vi "Inputs.vi"(8 "error in (no error)":errorcluster, 11 "State in":T1={"State"=enum."Idle", "Start Time"=timestamp(0 s since 1904-01-01), "Configuration"={"Cycle Period"=0.0, "Ismatech"={"VISA resource name"="", "Simulated?"=FALSE, "Pump Number"=1.0, "Reverse?"=FALSE}, "Masterflex"={"VISA resource name"="", "Simulated?"=FALSE, "Pump Number"=1.0, "Reverse?"=FALSE}, "Mettler"={"VISA resource name"="", "Simulated?"=FALSE}, "Bronkhorst M13 Flow Meter"={"VISA resource name"="", "Simulated?"=FALSE, "Smoothing Steps"=1}, "PID 2 Parameters"={"Input Device"=enum."Bronkhorst M13", "Output Device"=enum."Ismatec ISM 831C", "Setpoint"=0.0, "PID gains"={"proportional gain (Kc)"=1.0, "integral time (Ti, min)"=0.01, "derivative time (Td, min)"=0.0}}, "Manual Entry"=0.0, "Auto?"=TRUE, "PID range"={"PID High"=100.0, "PID Low"=0.0, "High Warning"=100.0}, "Tacmina Settings"={"Analog DAQ Task"="", "Digital DAQ Task"=""}, "KNF SIMDOS Settings"={"VISA resource name"="", "Simulated?"=TRUE}, "ASIA Pump C"={"ASIA Pump #"=0, "channel"=0, "Simulated"=FALSE}, "VICI Settings"={"VISA resource name"="", "Pump ID"="", "Pump Head Vol"=0.0, "Reverse?"=FALSE, "Simulated?"=FALSE}, "FLOM Settings"={"VISA resource name"="", "Simulated?"=TRUE, "Pump Number"=0.0}, "SSI PR/LD Settings"={"VISA resource name"="", "Simulated?"=FALSE}, "Masterflex 75211 Settings"={"Analog DAQ Task"="", "Digital DAQ Task"=""}, "SSI P40 Settings"={"VISA resource name"="", "Simulated?"=TRUE}, "Ismatech 3 Channel Settings"={"VISA resource name"="", "Pump Number"=1, "Channel Number"=0, "Simulated?"=TRUE, "Reverse?"=FALSE}, "Bronkhorst M14 Settings"={"VISA resource name"="", "Simulated?"=FALSE, "Smoothing Steps"=1}, "Reset Totalizer"=FALSE, "Input Num Alarm Settings"=[], "Control Type"=enum."g/min"}, "Current Time"=timestamp(0 s since 1904-01-01), "PID 1 Parameters"={"Setpoint"=0.0, "PID gains"={"proportional gain (Kc)"=1.0, "integral time (Ti, min)"=0.01, "derivative time (Td, min)"=0.0}}, "First Iteration"=FALSE, "Data"={"Flowmeter (g/min)"=0.0, "Flowmeter (ml/min)"=0.0, "Density"=0.0, "FL Temp"=0.0, "Scale Output (g)"=0.0, "Scale Rate of Change (g/min)"=0.0, "PID 1 Output"=0.0, "PID 2 Process Variable"=0.0, "PID 2 output"=0.0, "Pump Flow"=0.0, "Pump Pressure"=0.0, "Totalized Value"=0.0}, "Process Name"="", "Pump On?"=enum."Off", "Input Error"=FALSE, "Output Error"=FALSE, "Log Started"=FALSE, "PID Overshoot"=FALSE, "Current Setpoint"=0.0} {"PID 1 Parameters"."PID gains"."derivative time (Td, min)" format="%.3f"; "PID 1 Parameters"."PID gains"."integral time (Ti, min)" format="%.3f"; "PID 1 Parameters"."PID gains"."proportional gain (Kc)" format="%.3f"; "Configuration"."Bronkhorst M14 Settings"."Smoothing Steps" min=1 step=1; "Configuration"."Ismatech 3 Channel Settings"."Channel Number" min=0 max=3; "Configuration"."Ismatech 3 Channel Settings"."Pump Number" min=1; "Configuration"."PID range"."PID Low" min=0.0 max=100.0 format="%.2f"; "Configuration"."PID range"."PID High" format="%.2f"; "Configuration"."PID 2 Parameters"."PID gains"."derivative time (Td, min)" format="%.3f"; "Configuration"."PID 2 Parameters"."PID gains"."integral time (Ti, min)" format="%.3f"; "Configuration"."PID 2 Parameters"."PID gains"."proportional gain (Kc)" format="%.3f"; "Configuration"."Bronkhorst M13 Flow Meter"."Smoothing Steps" min=1 step=1; "Configuration"."ASIA Pump C"."channel" min=0 max=1 step=1; "Configuration"."Ismatech"."Pump Number" min=1.0 max=20.0 step=1.0; "Configuration"."Masterflex"."Pump Number" min=1.0 max=20.0 step=1.0}) -> (0 "error out":errorcluster, 3 "State out":T1={"State"=enum."Idle", "Start Time"=timestamp(0 s since 1904-01-01), "Configuration"={"Cycle Period"=0.0, "Ismatech"={"VISA resource name"="", "Simulated?"=FALSE, "Pump Number"=1.0, "Reverse?"=FALSE}, "Masterflex"={"VISA resource name"="", "Simulated?"=FALSE, "Pump Number"=1.0, "Reverse?"=FALSE}, "Mettler"={"VISA resource name"="", "Simulated?"=FALSE}, "Bronkhorst M13 Flow Meter"={"VISA resource name"="", "Simulated?"=FALSE, "Smoothing Steps"=1}, "PID 2 Parameters"={"Input Device"=enum."Bronkhorst M13", "Output Device"=enum."Ismatec ISM 831C", "Setpoint"=0.0, "PID gains"={"proportional gain (Kc)"=1.0, "integral time (Ti, min)"=0.01, "derivative time (Td, min)"=0.0}}, "Manual Entry"=0.0, "Auto?"=TRUE, "PID range"={"PID High"=100.0, "PID Low"=0.0, "High Warning"=100.0}, "Tacmina Settings"={"Analog DAQ Task"="", "Digital DAQ Task"=""}, "KNF SIMDOS Settings"={"VISA resource name"="", "Simulated?"=TRUE}, "ASIA Pump C"={"ASIA Pump #"=0, "channel"=0, "Simulated"=FALSE}, "VICI Settings"={"VISA resource name"="", "Pump ID"="", "Pump Head Vol"=0.0, "Reverse?"=FALSE, "Simulated?"=FALSE}, "FLOM Settings"={"VISA resource name"="", "Simulated?"=TRUE, "Pump Number"=0.0}, "SSI PR/LD Settings"={"VISA resource name"="", "Simulated?"=FALSE}, "Masterflex 75211 Settings"={"Analog DAQ Task"="", "Digital DAQ Task"=""}, "SSI P40 Settings"={"VISA resource name"="", "Simulated?"=TRUE}, "Ismatech 3 Channel Settings"={"VISA resource name"="", "Pump Number"=1, "Channel Number"=0, "Simulated?"=TRUE, "Reverse?"=FALSE}, "Bronkhorst M14 Settings"={"VISA resource name"="", "Simulated?"=FALSE, "Smoothing Steps"=1}, "Reset Totalizer"=FALSE, "Input Num Alarm Settings"=[], "Control Type"=enum."g/min"}, "Current Time"=timestamp(0 s since 1904-01-01), "PID 1 Parameters"={"Setpoint"=0.0, "PID gains"={"proportional gain (Kc)"=1.0, "integral time (Ti, min)"=0.01, "derivative time (Td, min)"=0.0}}, "First Iteration"=FALSE, "Data"={"Flowmeter (g/min)"=0.0, "Flowmeter (ml/min)"=0.0, "Density"=0.0, "FL Temp"=0.0, "Scale Output (g)"=0.0, "Scale Rate of Change (g/min)"=0.0, "PID 1 Output"=0.0, "PID 2 Process Variable"=0.0, "PID 2 output"=0.0, "Pump Flow"=0.0, "Pump Pressure"=0.0, "Totalized Value"=0.0}, "Process Name"="", "Pump On?"=enum."Off", "Input Error"=FALSE, "Output Error"=FALSE, "Log Started"=FALSE, "PID Overshoot"=FALSE, "Current Setpoint"=0.0} {"PID 1 Parameters"."PID gains"."derivative time (Td, min)" format="%.3f"; "PID 1 Parameters"."PID gains"."integral time (Ti, min)" format="%.3f"; "PID 1 Parameters"."PID gains"."proportional gain (Kc)" format="%.3f"; "Configuration"."Bronkhorst M14 Settings"."Smoothing Steps" min=1 step=1; "Configuration"."Ismatech 3 Channel Settings"."Channel Number" min=0 max=3; "Configuration"."Ismatech 3 Channel Settings"."Pump Number" min=1; "Configuration"."PID range"."PID Low" min=0.0 max=100.0 format="%.2f"; "Configuration"."PID range"."PID High" format="%.2f"; "Configuration"."PID 2 Parameters"."PID gains"."derivative time (Td, min)" format="%.3f"; "Configuration"."PID 2 Parameters"."PID gains"."integral time (Ti, min)" format="%.3f"; "Configuration"."PID 2 Parameters"."PID gains"."proportional gain (Kc)" format="%.3f"; "Configuration"."Bronkhorst M13 Flow Meter"."Smoothing Steps" min=1 step=1; "Configuration"."ASIA Pump C"."channel" min=0 max=1 step=1; "Configuration"."Ismatech"."Pump Number" min=1.0 max=20.0 step=1.0; "Configuration"."Masterflex"."Pump Number" min=1.0 max=20.0 step=1.0})   [LabVIEW 2018, in "Feed Module.lvlib" / "Feed Module Engine.lvlib"]
uses:
  Feed Module Engine.lvlib
  State Cluster.ctl
  State Enum.ctl
  Feed Module/Controls/Feed Module Settings Cluster.ctl
  Ismatec ISM 831C/Controls/Ismatech ISM831C Settings Cluster.ctl
  Masterflex 7550-30/Controls/Settings Cluster.ctl
  Mettler Toledo/Controls/Settings Cluster.ctl
  Bronkhorst M13 Flow Meter/Settings Cluster.ctl
  PID 2 Parameters Cluster.ctl
  PID Input Enum.ctl
  PID 2 Output Enum.ctl
  Tacmina QI/Tacmina QI DAQ Setting.ctl
  KNF Pump/Settings Cluster plus SIMDOS.ctl
  ASIA Pump/Pump Settings.ctl
  VICI M50 Party Mode/Settings Cluster.ctl
  FLOM Pump/Settings Cluster.ctl
  SSI PR Class/SSI PR or LD Settings Cluster.ctl
  Masterflex 75211/Masterflex 75211 DAQ Setting.ctl
  SSI PR Class/SSI P40 Settings Cluster.ctl
  Ismatec 78001/Ismatec 4083.ctl
  Bronkhorst M14 Flow Meter/Settings Cluster.ctl
  Tag VIs/Numeric Alarm Settings Cluster.ctl
  PID 1 Parameters Cluster.ctl
  Tag VIs/Tag FGV Operation Enum.ctl
  Mettler Toledo/Mettler Toledo.lvlib
  Bronkhorst M13 Flow Meter/Bronkhorst M13 Flow Meter.lvlib
  Shared Variables/Dynamic Shared Variables.lvlib
  Bronkhorst M14 Flow Meter/Bronkhorst M14 Flow Meter.lvlib
  Feed Module/Feed Module.lvlib
  Ismatec ISM 831C/Ismatec ISM 831C.lvlib
  Masterflex 7550-30/Masterflex 7550-30.lvlib
  Tacmina QI/Tacmina QI.lvlib
  KNF Pump/KNF SIMDOS.lvlib
  ASIA Pump.lvlib
  VICI M50 Party Mode/VICI M6 M50 Party Mode.lvlib
  FLOM Pump/FLOM Pump.lvlib
  SSI PR Class/SSI PR or LD Pump.lvlib
  Masterflex 75211/Masterflex 75211.lvlib
  SSI PR Class/SSI P40 Pump.lvlib
  Ismatec 78001/Ismatec 4308.lvlib
panel:
  # "Output Instruments"
  # "Input Instruments"
  # "Output Instruments"
  # "Input Instruments"
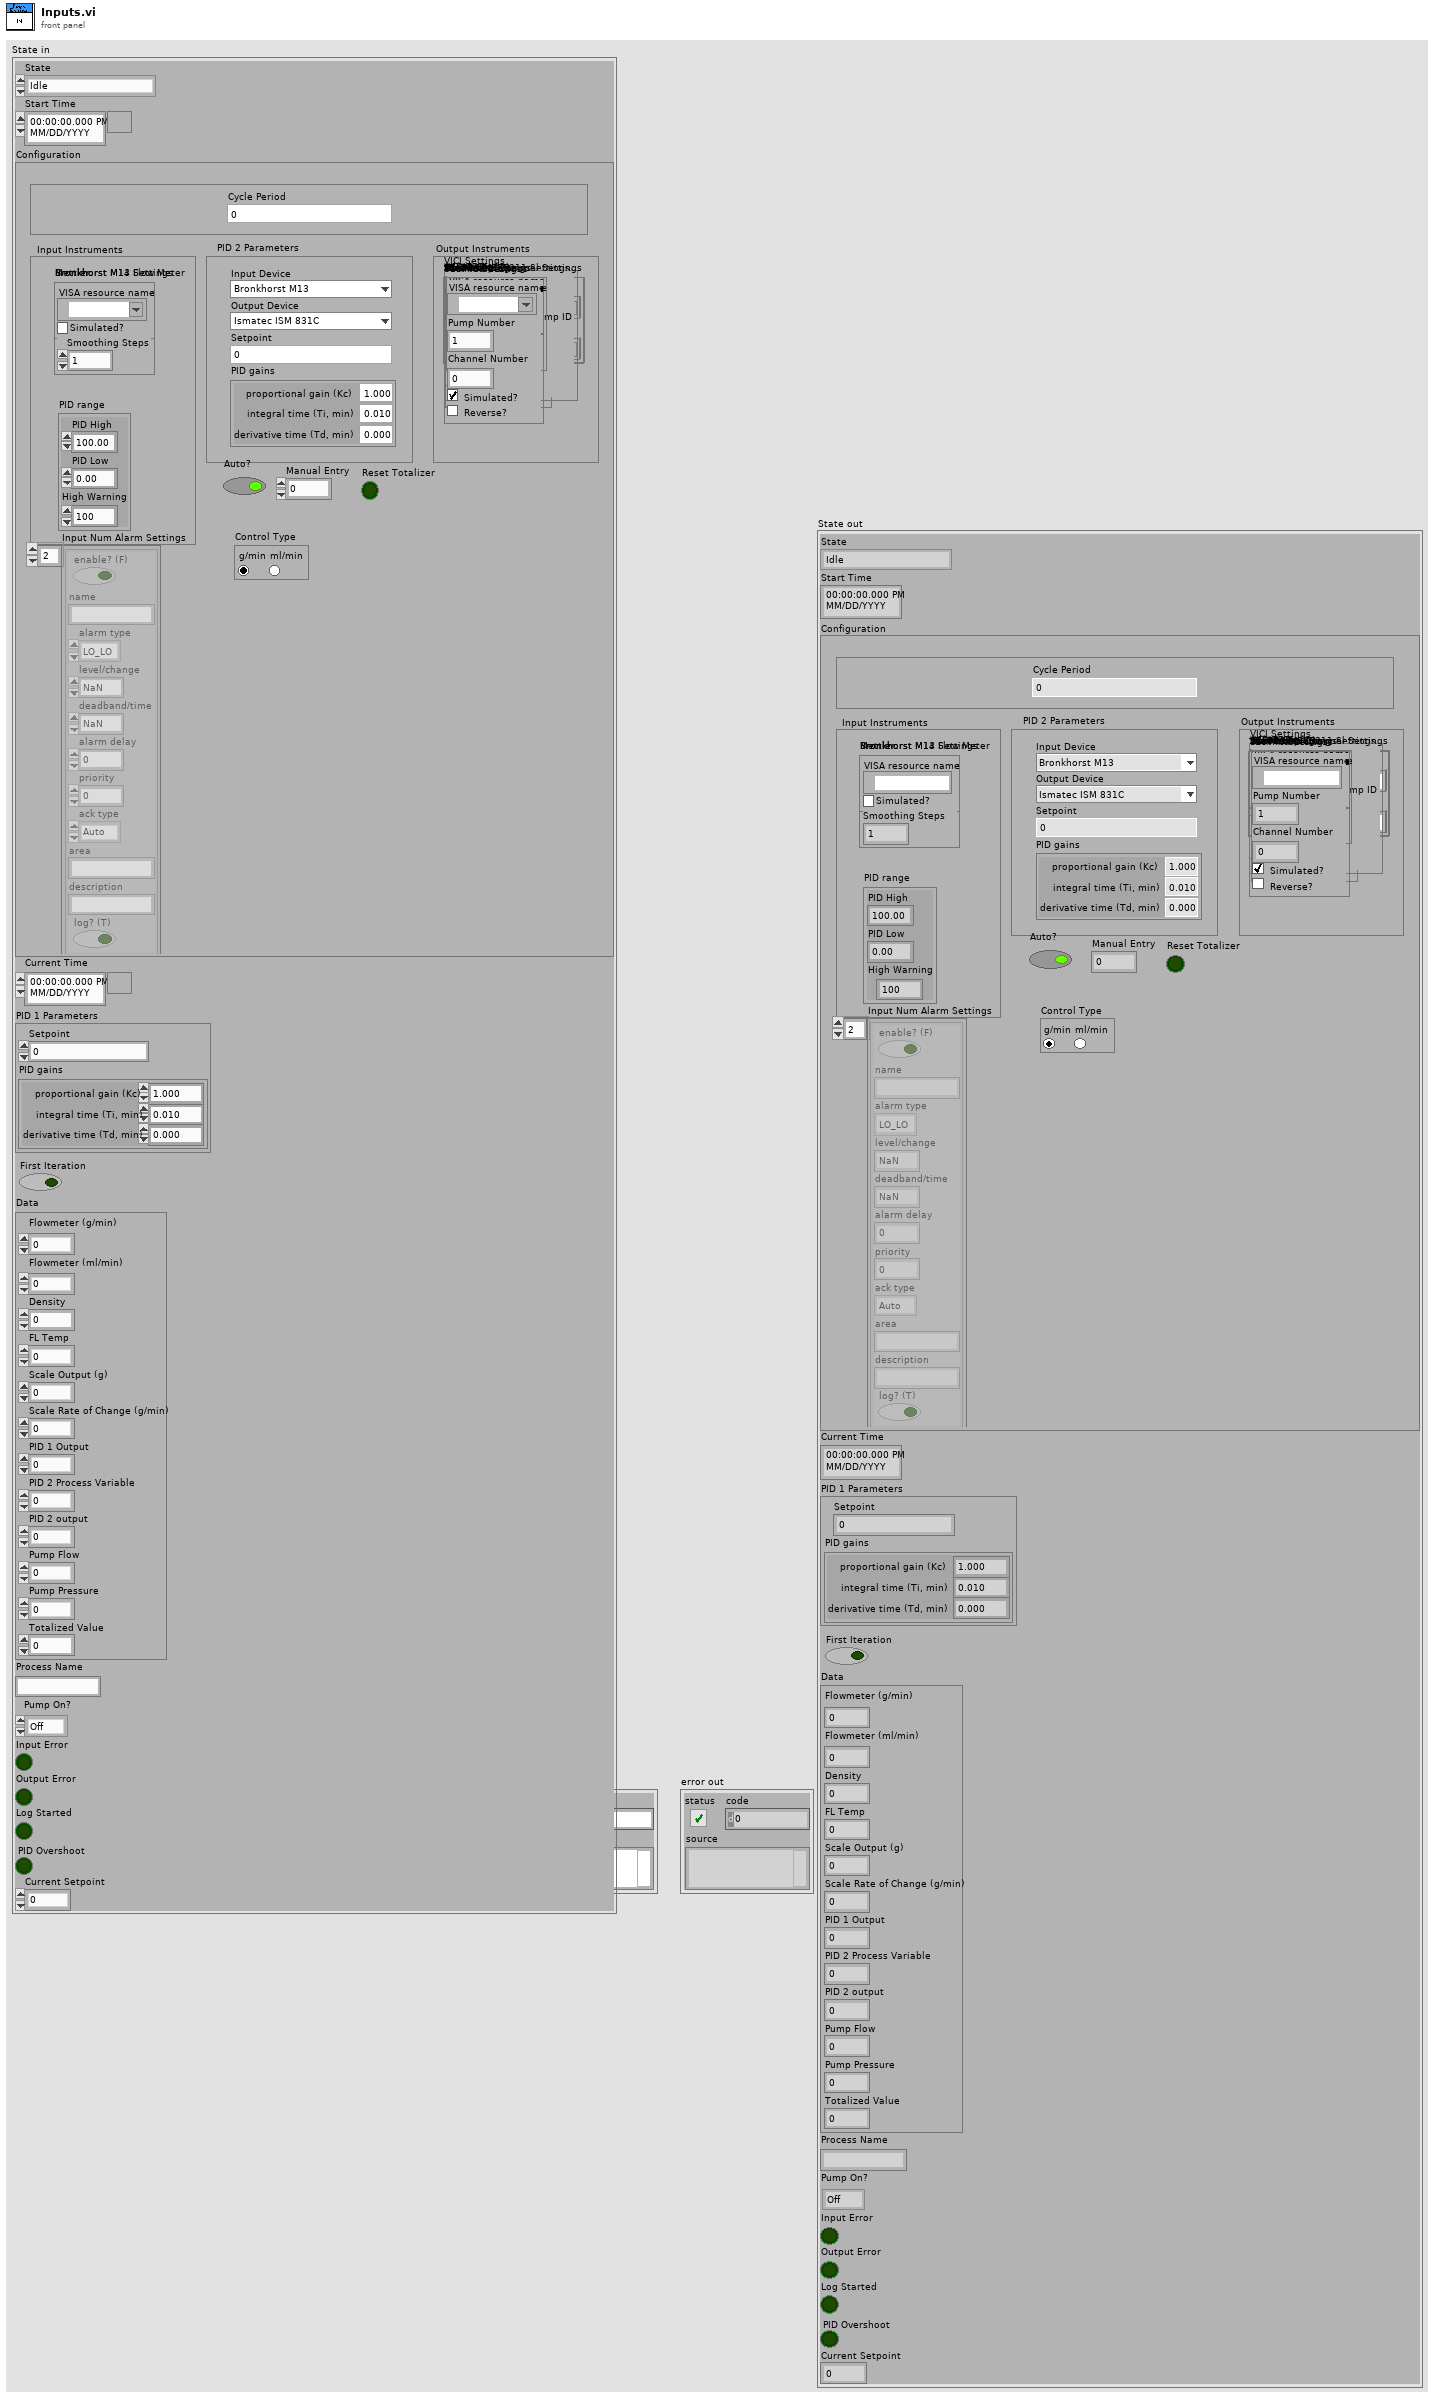
[diagram p1: front panel]
types:
  T1 = typedef "Feed Module.lvlib/Feed Module Engine.lvlib/State Cluster.ctl" = cluster{"State":T2, "Start Time":timestamp, "Configuration":T3, "Current Time":timestamp, "PID 1 Parameters":T22, "First Iteration":bool, "Data":cluster{"Flowmeter (g/min)":dbl, "Flowmeter (ml/min)":dbl, "Density":dbl, "FL Temp":dbl, "Scale Output (g)":dbl, "Scale Rate of Change (g/min)":dbl, "PID 1 Output":dbl, "PID 2 Process Variable":dbl, "PID 2 output":dbl, "Pump Flow":dbl, "Pump Pressure":dbl, "Totalized Value":dbl}, "Process Name":string, "Pump On?":enum16{"Off", "On", "Not Initialized"}, "Input Error":bool, "Output Error":bool, "Log Started":bool, "PID Overshoot":bool, "Current Setpoint":dbl}
  T2 = typedef "Feed Module.lvlib/Feed Module Engine.lvlib/State Enum.ctl" = enum16{"Measuring", "Idle", "Paused"}
  T3 = typedef "Feed Module.lvlib/Feed Module Settings Cluster.ctl" = cluster{"Cycle Period":dbl, "Ismatech":T4, "Masterflex":T5, "Mettler":T6, "Bronkhorst M13 Flow Meter":T7, "PID 2 Parameters":T8, "Manual Entry":dbl, "Auto?":bool, "PID range":cluster{"PID High":dbl, "PID Low":dbl, "High Warning":dbl}, "Tacmina Settings":T11, "KNF SIMDOS Settings":T12, "ASIA Pump C":T13, "VICI Settings":T14, "FLOM Settings":T15, "SSI PR/LD Settings":T16, "Masterflex 75211 Settings":T17, "SSI P40 Settings":T18, "Ismatech 3 Channel Settings":T19, "Bronkhorst M14 Settings":T20, "Reset Totalizer":bool, "Input Num Alarm Settings":T21[], "Control Type":enum32{"g/min", "ml/min"}}
  T4 = typedef "Ismatec ISM 831C.lvlib/Ismatech ISM831C Settings Cluster.ctl" = cluster{"VISA resource name":refnum<visa-resource-name>, "Simulated?":bool, "Pump Number":dbl, "Reverse?":bool}
  T5 = typedef "Masterflex 7550-30.lvlib/Settings Cluster.ctl" = cluster{"VISA resource name":refnum<visa-resource-name>, "Simulated?":bool, "Pump Number":dbl, "Reverse?":bool}
  T6 = typedef "Mettler Toledo.lvlib/Settings Cluster.ctl" = cluster{"VISA resource name":refnum<visa-resource-name>, "Simulated?":bool}
  T7 = typedef "Bronkhorst M13 Flow Meter.lvlib/Settings Cluster.ctl" = cluster{"VISA resource name":refnum<visa-resource-name>, "Simulated?":bool, "Smoothing Steps":i32}
  T8 = typedef "PID 2 Parameters Cluster.ctl" = cluster{"Input Device":T9, "Output Device":T10, "Setpoint":dbl, "PID gains":cluster{"proportional gain (Kc)":dbl, "integral time (Ti, min)":dbl, "derivative time (Td, min)":dbl}}
  T9 = typedef "PID Input Enum.ctl" = enum16{"Default", "Bronkhorst M13", "Bronkhorst M14", "Scale Rate of Change"}
  T10 = typedef "PID 2 Output Enum.ctl" = enum16{"Default", "Ismatec ISM 4308", "Ismatec ISM 831C", "Masterflex 7550-30", "VICI M6", "VICI M50", "Tacmina QI", "KNF SIMDOS", "ASIA Type C", "FLOM UI-22-11", "SSI PR/LD", "SSI P40", "Masterflex 75211-70"}
  T11 = typedef "Tacmina QI.lvlib/Tacmina QI DAQ Setting.ctl" = cluster{"Analog DAQ Task":refnum<k21>, "Digital DAQ Task":refnum<k21>}
  T12 = typedef "KNF SIMDOS.lvlib/Settings Cluster plus SIMDOS.ctl" = cluster{"VISA resource name":refnum<visa-resource-name>, "Simulated?":bool}
  T13 = typedef "ASIA Pump.lvlib/Pump Settings.ctl" = cluster{"ASIA Pump #":i32, "channel":i32, "Simulated":bool}
  T14 = typedef "VICI M6 M50 Party Mode.lvlib/Settings Cluster.ctl" = cluster{"VISA resource name":refnum<visa-resource-name>, "Pump ID":string, "Pump Head Vol":dbl, "Reverse?":bool, "Simulated?":bool}
  T15 = typedef "FLOM Pump.lvlib/Settings Cluster.ctl" = cluster{"VISA resource name":refnum<visa-resource-name>, "Simulated?":bool, "Pump Number":dbl}
  T16 = typedef "SSI PR or LD Pump.lvlib/SSI PR or LD Settings Cluster.ctl" = cluster{"VISA resource name":refnum<visa-resource-name>, "Simulated?":bool}
  T17 = typedef "Masterflex 75211.lvlib/Masterflex 75211 DAQ Setting.ctl" = cluster{"Analog DAQ Task":refnum<k21>, "Digital DAQ Task":refnum<k21>}
  T18 = typedef "SSI P40 Pump.lvlib/SSI P40 Settings Cluster.ctl" = cluster{"VISA resource name":refnum<visa-resource-name>, "Simulated?":bool}
  T19 = typedef "Ismatec 4308.lvlib/Ismatec 4083.ctl" = cluster{"VISA resource name":refnum<visa-resource-name>, "Pump Number":i16, "Channel Number":i16, "Simulated?":bool, "Reverse?":bool}
  T20 = typedef "Bronkhorst M14 Flow Meter.lvlib/Settings Cluster.ctl" = cluster{"VISA resource name":refnum<visa-resource-name>, "Simulated?":bool, "Smoothing Steps":i32}
  T21 = typedef "Numeric Alarm Settings Cluster.ctl" = cluster{"enable? (F)":bool, "name":string, "alarm type":enum16{"HI_HI", "HI", "LO", "LO_LO"}, "level/change":dbl, "deadband/time":dbl, "alarm delay":dbl, "priority":u32, "ack type":enum16{"Auto", "User", "None", "Each Occurrence"}, "area":string, "description":string, "log? (T)":bool}
  T22 = typedef "PID 1 Parameters Cluster.ctl" = cluster{"Setpoint":dbl, "PID gains":cluster{"proportional gain (Kc)":dbl, "integral time (Ti, min)":dbl, "derivative time (Td, min)":dbl}}
  T23 = typedef "Tag FGV Operation Enum.ctl" = enum16{"Init", "Set Notification Queue", "Create Tag", "Commit", "Write Tag (Numeric)", "Write Tag (Boolean)", "Read All Tags", "Read One Tag", "Delete Tag Category", "Set Alarm Parameters (Numeric)", "Set Alarm Parameters (Boolean)", "Enable All Alarms", "Disable All Alarms", "Delete All Tags", "Read Alarms", "Ack Alarm", "Read Alarm Parameters (Numeric)", "Read Alarm Parameters (Boolean)"}
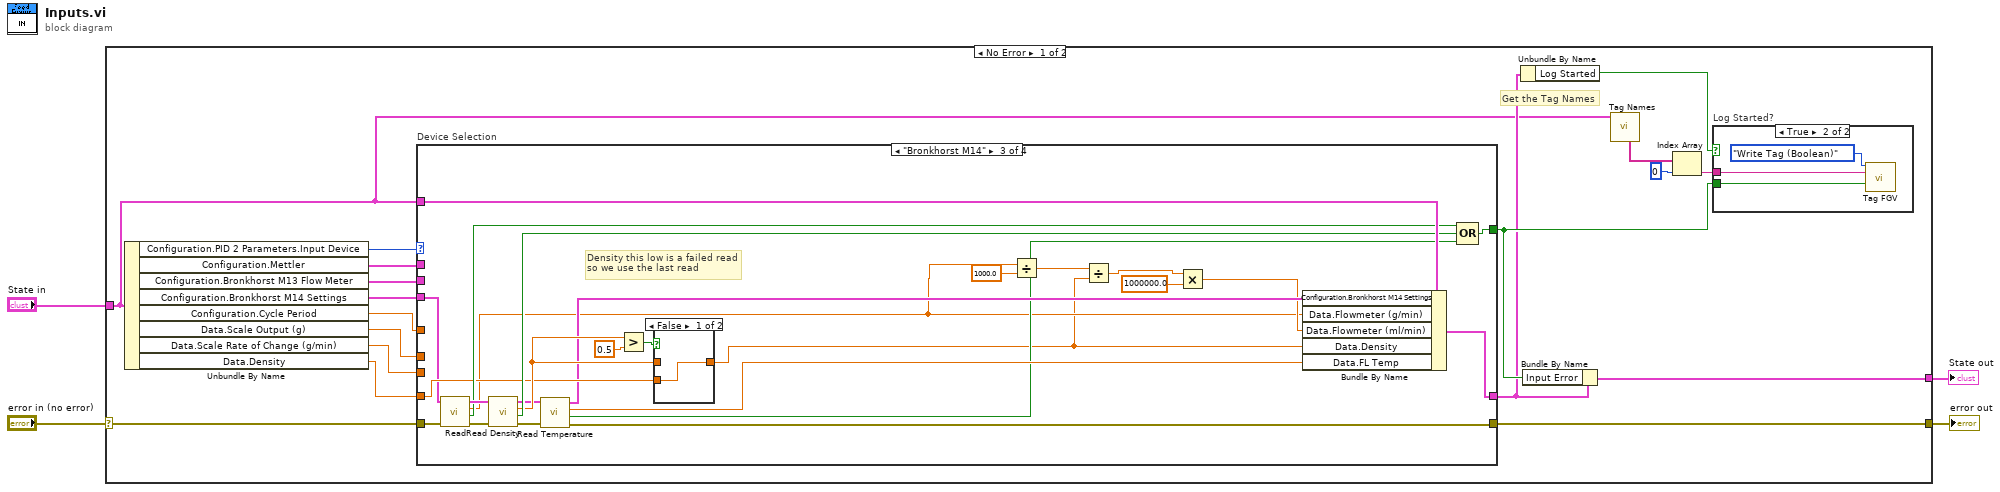
[diagram p0: block diagram]
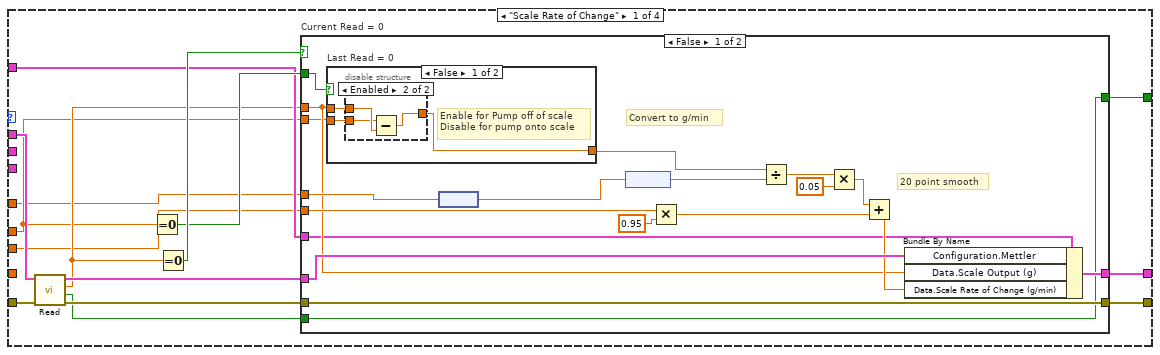
[diagram p3: hidden frame]
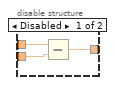
[diagram p4: hidden frame]
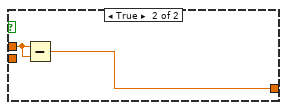
[diagram p5: hidden frame]
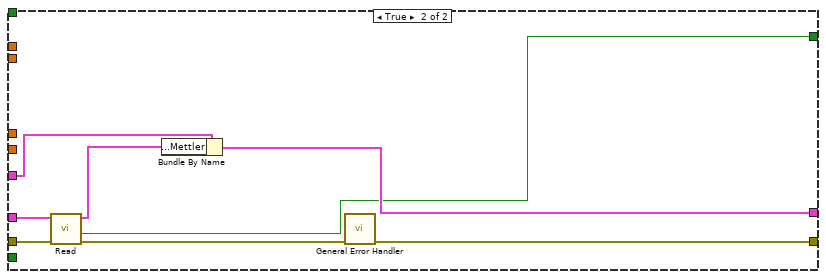
[diagram p6: hidden frame]
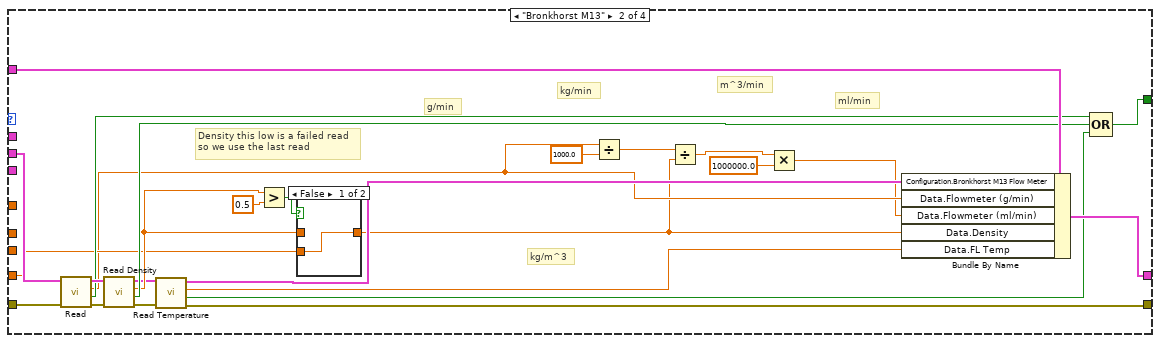
[diagram p7: hidden frame]
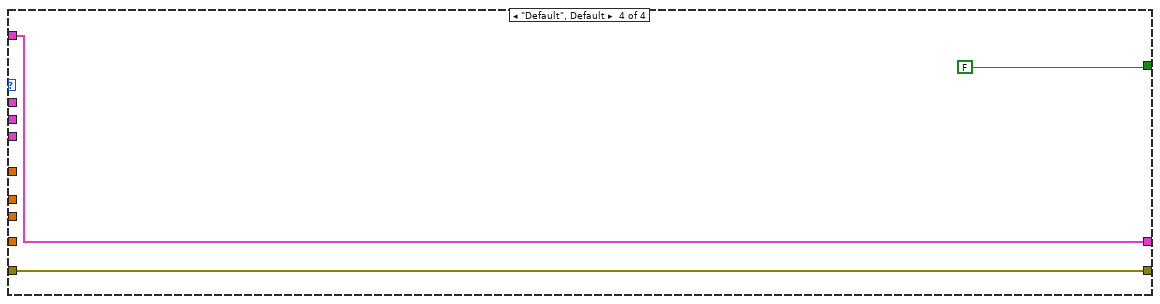
[diagram p10: hidden frame]
diagram:
  n1 = case shown="No Error" "error in (no error)" {
    selector: "error in (no error)" -> [w19 w138]
    tunnel: [w16 w138] -> w1
    tunnel: "State in" -> [w10 w137]
    tunnel: [w14 w137] -> w2
    frame No Error {
      # "Get the Tag Names"
      n2 = Unbundle By Name(w10) -> ("Configuration.PID 2 Parameters.Input Device"=w22:T9, "Configuration.Mettler"=w21:T6, "Configuration.Bronkhorst M13 Flow Meter"=w20:T7, "Configuration.Bronkhorst M14 Settings"=w8:T20, "Configuration.Cycle Period"=w9:dbl, "Data.Scale Output (g)"=w18:dbl, "Data.Scale Rate of Change (g/min)"=w17:dbl, "Data.Density"=w13:dbl)
      n3 = case "Device Selection" shown="\"Bronkhorst M14\"" w22 {
        tunnel: w10 -> [w35 w103 w131 w136]
        tunnel: [w31 w102 w130 w136] -> w12
        tunnel: w21 -> [w39 _ _ _]
        tunnel: w20 -> [_ w100 _ _]
        tunnel: w9 -> [w32 _ _ _]
        tunnel: w19 -> [w40 w101 w129 w135]
        tunnel: [w29 w87 w116 w135] -> w16
        tunnel: w18 -> [w33 _ _ _]
        tunnel: w17 -> [w28 _ _ _]
        tunnel: [w27 w95 w124 FALSE ("Connection Error")] -> w15
        tunnel: w13 -> [_ w91 w120 _]
        tunnel: w8 -> [_ _ w113 _]
        frame "Scale Rate of Change" {
          n4 = call "Read.vi"("error in (no error)"=w40, "Mettler Settings in"=w39) -> ("error out"=w30:errorcluster, "Connection Error"=w26:bool, "mass (g)"=w34:dbl, "Mettler Settings out"=w36:T6)  [unwired: 6 in]
          n5 = Equal To 0?(x=w33) -> (x = 0?=w37:bool)
          n6 = Equal To 0?(x=w34) -> (x = 0?=w38:bool)
          n7 = case "Current Read = 0" shown="False" w38 {
            tunnel: w34 -> [w44 _]
            tunnel: w33 -> [w43 _]
            tunnel: w35 -> [w41 w74]
            tunnel: w36 -> [w59 w77]
            tunnel: [w58 w72] -> w31
            tunnel: w32 -> [w55 _]
            tunnel: w37 -> [w53 _]
            tunnel: w30 -> [w52 w75]
            tunnel: [w52 w73] -> w29
            tunnel: w28 -> [w45 _]
            tunnel: [w42 w71] -> w27
            tunnel: w26 -> [w42 _]
            frame False {
              # "20 point smooth"
              # "Convert to g/min"
              n8 = case "Last Read = 0" shown="False" w53 {
                tunnel: [w61 w70] -> w57
                tunnel: w44 -> [w60 w69]
                tunnel: w43 -> [w62 _]
                frame False {
                  # "Enable for Pump off of scale\nDisable for pump onto scale"
                  n9 = disable-structure shown="Enabled" {
                    disable-tunnel: w62 -> [w65 w67]
                    disable-tunnel: w60 -> [w64 w68]
                    disable-tunnel: [w63 w66] -> w61
                    frame Disabled {
                      n10 = Subtract(x=w64, y=w65) -> (x-y=w63:dbl)
                    }
                    frame Enabled {
                      n11 = Subtract(x=w67, y=w68) -> (x-y=w66:dbl)
                    }
                  }
                }
                frame True {
                  n12 = Subtract(x=w69, y=w69) -> (x-y=w70:dbl)
                }
              }
              n13 = node(w55) -> (w54:dbl[unit])
              n14 = node(w54) -> (w56:dbl)
              n15 = Multiply(x=w45, y=0.95) -> (x*y=w51:dbl)
              n16 = Divide(x=w57, y=w56) -> (x/y=w47:dbl)
              n17 = Multiply(x=w47, y=0.05) -> (x*y=w48:dbl)
              n18 = Add(x=w48, y=w51) -> (x+y=w46:dbl)
              n19 = Bundle By Name(cluster=w41, "Configuration.Mettler"=w59, "Data.Scale Output (g)"=w44, "Data.Scale Rate of Change (g/min)"=w46) -> (w58:T1)
            }
            frame True {
              n20 = call "Read.vi"("error in (no error)"=w75, "Mettler Settings in"=w77) -> ("error out"=w73:errorcluster, "Connection Error"=w71:bool, "Mettler Settings out"=w76:T6)  [unwired: 6 in, 1 out]
              n21 = Bundle By Name(cluster=w74, "Configuration.Mettler"=w76) -> (w72:T1)
              n22 = call <vilib>:"General Error Handler.vi"("error in (no error)"=w73) -> ()  [unwired: 10 in, 5 out]
            }
          }
        }
        frame "Bronkhorst M13" {
          # "g/min"
          # "ml/min"
          # "m^3/min"
          # "kg/m^3"
          # "kg/min"
          # "Density this low is a failed read\nso we use the last read"
          n23 = call "Read.vi"("error in (no error)"=w101, "Bronkhorst Settings in"=w100) -> ("error out"=w99:errorcluster, "Connection Error"=w97:bool, "flow"=w83:dbl, "Bronkhorst Settings out"=w98:T7)  [unwired: 6 in]
          n24 = call "Read Density.vi"("error in (no error)"=w99, "Bronkhorst Settings in"=w98) -> ("error out"=w90:errorcluster, "Connection Error"=w96:bool, "Density kg/m^3"=w92:sgl, "Bronkhorst Settings out"=w89:T7)  [unwired: 6 in]
          n25 = call "Read Temperature.vi"("error in (no error)"=w90, "Bronkhorst Settings in"=w89) -> ("error out"=w87:errorcluster, "Connection Error"=w85:bool, "Temp (C)"=w86:sgl, "Bronkhorst Settings out"=w88:T7)  [unwired: 6 in]
          n26 = Greater?(x=w92, y=sgl 0.5) -> (0:w94:bool)
          n27 = case shown="False" w94 {
            tunnel: w92 -> [_ w105]
            tunnel: [w104 w105] -> w81
            tunnel: w91 -> [w104 _]
            frame False {
            }
            frame True {
            }
          }
          n28 = Divide(x=w83, y=1000.0) -> (x/y=w82:dbl)
          n29 = Divide(x=w82, y=w81) -> (x/y=w79:dbl)
          n30 = Multiply(x=w79, y=1000000.0) -> (x*y=w78:dbl)
          n31 = Bundle By Name(cluster=w103, "Configuration.Bronkhorst M13 Flow Meter"=w88, "Data.Flowmeter (g/min)"=w83, "Data.Flowmeter (ml/min)"=w78, "Data.Density"=w81, "Data.FL Temp"=w86) -> (w102:T1)
          n32 = Compound Arithmetic op=OR(w97, w96, w85) -> (w95:bool)
        }
        frame "Bronkhorst M14" {
          # "Density this low is a failed read\nso we use the last read"
          n33 = call "Read.vi"("error in (no error)"=w129, "Bronkhorst Settings in"=w113) -> ("error out"=w128:errorcluster, "Connection Error"=w126:bool, "flow"=w107:dbl, "Bronkhorst Settings out"=w127:T20)  [unwired: 6 in]
          n34 = call "Read Density.vi"("error in (no error)"=w128, "Bronkhorst Settings in"=w127) -> ("error out"=w119:errorcluster, "Connection Error"=w125:bool, "Density kg/m^3"=w121:sgl, "Bronkhorst Settings out"=w118:T7)  [unwired: 6 in]
          n35 = call "Read Temperature.vi"("error in (no error)"=w119, "Bronkhorst Settings in"=w118) -> ("error out"=w116:errorcluster, "Connection Error"=w114:bool, "Temp (C)"=w115:sgl, "Bronkhorst Settings out"=w117:T7)  [unwired: 6 in]
          n36 = Greater?(x=w121, y=sgl 0.5) -> (0:w123:bool)
          n37 = case shown="False" w123 {
            tunnel: w121 -> [_ w133]
            tunnel: [w132 w133] -> w106
            tunnel: w120 -> [w132 _]
            frame False {
            }
            frame True {
            }
          }
          n38 = Divide(x=w107, y=1000.0) -> (x/y=w111:dbl)
          n39 = Divide(x=w111, y=w106) -> (x/y=w109:dbl)
          n40 = Multiply(x=w109, y=1000000.0) -> (x*y=w108:dbl)
          n41 = Bundle By Name(cluster=w131, "Configuration.Bronkhorst M14 Settings"=w117, "Data.Flowmeter (g/min)"=w107, "Data.Flowmeter (ml/min)"=w108, "Data.Density"=w106, "Data.FL Temp"=w115) -> (w130:T1)
          n42 = Compound Arithmetic op=OR(w126, w125, w114) -> (w124:bool)
        }
        frame "Default", Default {
        }
      }
      n43 = Unbundle By Name(w12) -> ("Log Started"=w11:bool)
      n44 = Bundle By Name(cluster=w12, "Input Error"=w15) -> (w14:T1)
      n45 = call "Tag Names.vi"("State in"=w10) -> ("All Boolean Tags"=w7:string[])  [unwired: 6 in, 4 out]
      n46 = Index Array(array=w7, index=0) -> (element=w5:string)
      n47 = case "Log Started?" shown="True" w11 {
        tunnel: w5 -> [_ w25]
        tunnel: w15 -> [_ w23]
        frame False {
        }
        frame True {
          n48 = call "Tag FGV.vi"("Operation"=Tag_FGV_Operation_Enum."Write Tag (Boolean)", "Tag Name"=w25, "Data"=w23) -> ()  [unwired: 5 in, 8 out]
        }
      }
    }
    frame Error {
    }
  }
  "error out" <- w1
  "State out" <- w2
